vi "setDigitalOutput.vi"(3 "error in":errorcluster, 4 "data":bool[](array[boolean])=[FALSE, FALSE, FALSE, FALSE, FALSE, FALSE, TRUE, TRUE], 5 "Line(s)":tag="Dev8/port0/line0:7") -> (0 "error out":errorcluster)   [LabVIEW 2016]
uses:
  <vilib>/DAQmx/write.llb/DAQmx Write (Digital 1D Bool 1Chan 1Samp).vi
  <vilib>/DAQmx/create/channels.llb/DAQmx Create Channel (DO-Digital Output).vi
  <vilib>/DAQmx/miscellaneous.llb/DAQmx Fill In Error Info.vi
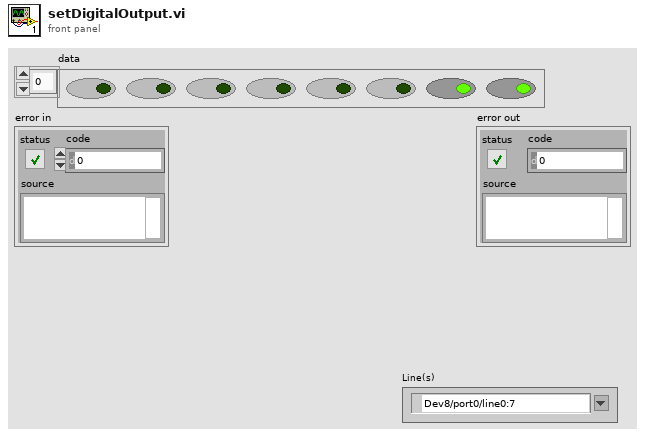
[diagram p1: front panel]
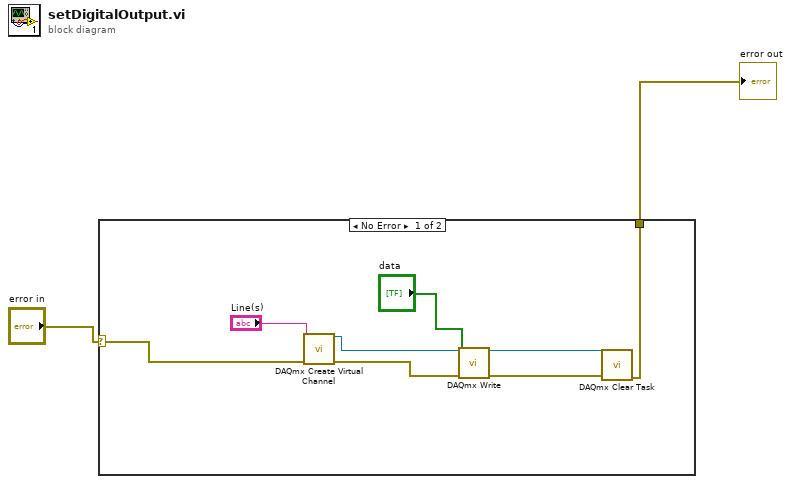
[diagram p0: block diagram]
diagram:
  n1 = case shown="No Error" "error in" {
    selector: "error in" -> [w4 w11]
    tunnel: [w3 w11] -> w1
    frame No Error {
      n2 = call-poly <vilib>:"DAQmx Create Virtual Channel.vi"("lines"="Line(s)", "error in"=w4) -> ("task out"=w6:refnum<k21>, "error out"=w8:errorcluster)  [unwired: 12 in]
      n3 = call-poly <vilib>:"DAQmx Write.vi"("task/channels in"=w6, "data"="data", "error in"=w8) -> ("task out"=w7:refnum<k21>, "error out"=w9:errorcluster)  [unwired: 10 in, 1 out]
      n4 = call <vilib>:"DAQmx Clear Task.vi"("task in"=w7, "error in"=w9) -> ("error out"=w3:errorcluster)  [unwired: 13 in]
    }
    frame Error {
    }
  }
  "error out" <- w1
